vi "Fit.vi"(7 "Type X":T1(ring), 8 "error in (no error)":errorcluster caption="entrée d'erreur (pas d'erreur)", 9 "y":string[][](array[string]), 10 "X":string[][](array[string]), 11 "TfidfTransformer.lvclass":refnum<class "TfidfTransformer.lvclass">) -> (0 "error out":errorcluster caption="sortie d'erreur", 2 "String Data":string, 3 "TfidfTransformer.lvclass":refnum<class "TfidfTransformer.lvclass">)   [LabVIEW 2020, in "TfidfTransformer.lvclass"]
doc: "Learn the idf vector (global term weights).\n\nReturns :\n\n- String : OK"
uses:
  TfidfTransformer.lvclass
  TfidfTransformer.lvclass/TfidfTransformer.ctl
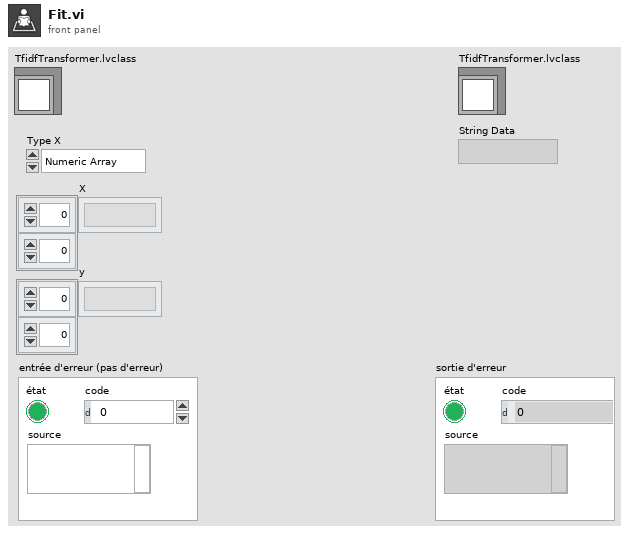
[diagram p1: front panel]
types:
  T1 = enum16{"Numeric Array", "String Array", "Sparse"}
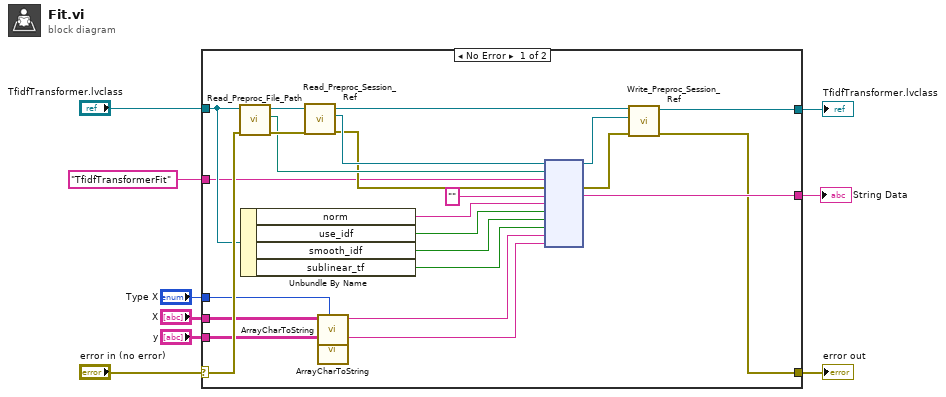
[diagram p0: block diagram]
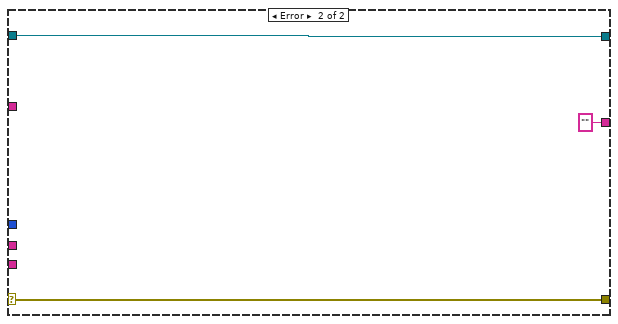
[diagram p2: hidden frame]
diagram:
  n1 = case shown="No Error" "error in (no error)" {
    selector: "error in (no error)" -> [w24 w36]
    tunnel: [w10 w36] -> w8
    tunnel: [w11 w35] -> w6
    tunnel: "TfidfTransformer.lvclass" -> [w23 w35]
    tunnel: "TfidfTransformerFit" ("Fonction") -> [w22 _]
    tunnel: [w21 ""] -> w4
    tunnel: "X" -> [w16 _]
    tunnel: "y" -> [w15 _]
    tunnel: "Type X" -> [w12 _]
    frame No Error {
      n2 = call-dynamic "Read_Preproc_File_Path.vi"("error in (no error)"=w24, "Python in"=w23) -> ("error out"=w32:errorcluster, "File_Path"=w31:path, "Python out"=w33:refnum<class "TfidfTransformer.lvclass">)  [unwired: 7 in]
      n3 = Unbundle By Name(w23) -> ("norm"=w20:string, "use_idf"=w19:bool, "smooth_idf"=w18:bool, "sublinear_tf"=w17:bool)
      n4 = call-dynamic "Read_Preproc_Session_Ref.vi"("error in (no error)"=w32, "Python in"=w33) -> ("error out"=w29:errorcluster, "Session_ref"=w30:refnum<k35>, "Python out"=w28:refnum<class "TfidfTransformer.lvclass">)  [unwired: 7 in]
      n5 = call "ArrayCharToString.vi"("Type"=w12, "TAB"=w16) -> ("Instruction"=w14:string)  [unwired: 9 in]
      n6 = call "ArrayCharToString.vi"("TAB"=w15) -> ("Instruction"=w13:string)  [unwired: 10 in]
      n7 = node(w30, w31, w22, w29, "", w20, w19, w18, w17, w14, w13) -> (w26:refnum<k35>, w27:errorcluster, w21:string)  [unwired: 6 in, 2 out]
      n8 = call-dynamic "Write_Preproc_Session_Ref.vi"("error in (no error)"=w27, "Session_ref"=w26, "Python in"=w28) -> ("error out"=w10:errorcluster, "Python out"=w11:refnum<class "TfidfTransformer.lvclass">)  [unwired: 7 in]
    }
    frame Error {
    }
  }
  "error out" <- w8
  "TfidfTransformer.lvclass" <- w6
  "String Data" <- w4
